vi "VI Close Function.vi"(10 "Stop In":bool) -> (2 "Stop out":bool)   [LabVIEW 2021]
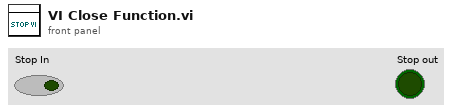
[diagram p1: front panel]
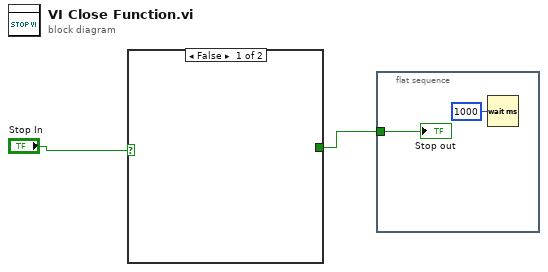
[diagram p0: block diagram]
diagram:
  n1 = case shown="False" "Stop In" {
    selector: "Stop In" -> [_ w3]
    tunnel: [_ w3] -> w1
    frame False {
    }
    frame True {
    }
  }
  n2 = flat-sequence {
    tunnel: w1 -> [w5]
    frame #0 {
      n3 = Wait (ms)(milliseconds to wait=u32 1000) -> ()  [unwired: 1 out]
      "Stop out" <- w5
    }
  }
